vi "Generate_I2C.vi"(8 "Error_In":errorcluster, 10 "Mode":T1, 11 "7Bit_Address_In":refnum<class "7Bit_Address.lvclass">) -> (0 "Error_Out":errorcluster, 3 "7Bit_Address_Out":refnum<class "7Bit_Address.lvclass">)   [LabVIEW 2023, in "7Bit_Address.lvclass"]
uses:
  7Bit_Address.lvclass
  D:/Git/Assignments/SDLC_I2C/SDLC_I2C_LV23V/Class/I2C/I2C.lvclass
  Class/I2C/Controls/Mode.ctl
  Controls/I2C_States.ctl
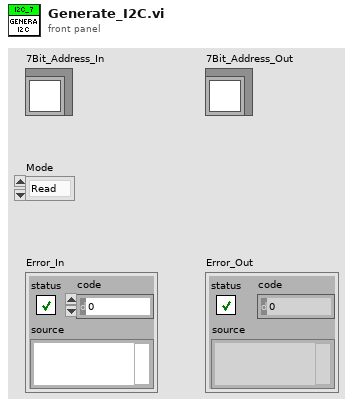
[diagram p1: front panel]
types:
  T1 = typedef "Mode.ctl" = enum16{"Read", "Write"}
  T2 = typedef "I2C_States.ctl" = enum16{"Start", "Byte", "Ack_Nack", "Stop"}
  T3 = typedef "Converted_Data.ctl" = cluster{"Vmin":dbl, "Vmax":dbl, "Input":string, "Off_Set (uS)":dbl, "T_HD_STA (uS)":dbl, "Sample_Per_Us":dbl, "T_HD_DAT (uS)":dbl, "T_SU_DAT (uS)":dbl, "Frequency (kHz)":dbl, "T_SU_STO":dbl, "T_Off (uS)":dbl, "T_On (uS)":dbl, "T_BUF":dbl, "Target_Address":u16, "Register_Address":u8, "Byte_Array":u8[]}
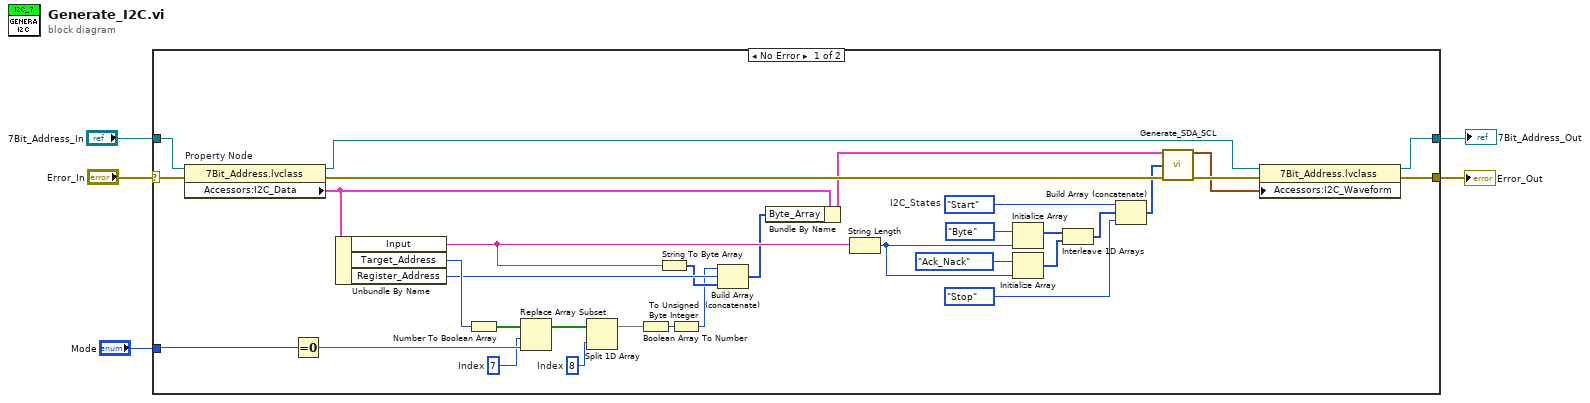
[diagram p0: block diagram]
diagram:
  n1 = case shown="No Error" "Error_In" {
    selector: "Error_In" -> [w37 w40]
    tunnel: [w9 w40] -> w5
    tunnel: [w11 w39] -> w4
    tunnel: "7Bit_Address_In" -> [w26 w39]
    tunnel: "Mode" -> [w22 _]
    frame No Error {
      w6 = 8  # Index
      w19 = 7  # Index
      w35 = I2C_States."Start"  # I2C_States
      n2 = property on="Property Node" class="7Bit_Address.lvclass"(reference=w26, error in=w37) -> (reference out=w25:refnum<class "7Bit_Address.lvclass">, error out=w36:errorcluster, "Accessors:I2C_Data"=w10:T3)
      n3 = Equal To 0?(x=w22) -> (x = 0?=w20:bool)
      n4 = Unbundle By Name(w10) -> ("Input"=w23:string, "Target_Address"=w18:u16, "Register_Address"=w16:u8)
      n5 = Number To Boolean Array(number=w18) -> (Boolean array=w21:bool[])
      n6 = Replace Array Subset(array=w21, new element=w20, index=w19) -> (w8:bool[])
      n7 = Split 1D Array(array=w8, index=w6) -> (first subarray=w7:bool[])  [unwired: 1 out]
      n8 = Boolean Array To Number(Boolean array=w7) -> (number=w17:u32)
      n9 = String To Byte Array(string=w23) -> (unsigned byte array=w15:u8[])
      n10 = To Unsigned Byte Integer(number=w17) -> (unsigned 8bit integer=w14:u8)
      n11 = Build Array (concatenate)(w14, w16, w15) -> (w12:u8[])
      n12 = Bundle By Name(cluster=w10, "Byte_Array"=w12) -> (w13:T3)
      n13 = String Length(string=w23) -> (length=w33:i32)
      n14 = Initialize Array(I2C_States."Byte" ("Enum"), w33) -> (w31:T2[])
      n15 = Initialize Array(I2C_States."Ack_Nack" ("element"), w33) -> (w30:T2[])
      n16 = Interleave 1D Arrays(w31, w30) -> (w29:T2[])
      n17 = Build Array (concatenate)(w35, w29, I2C_States."Stop" ("element")) -> (w27:T2[])
      n18 = call "Generate_SDA_SCL.vi"("Data"=w13, "Data_Sequence"=w27, "Error_In"=w36) -> ("Waveform Graph"=w24:waveform(dbl)[], "Error_Out"=w38:errorcluster)  [unwired: 11 in]
      n19 = property class="7Bit_Address.lvclass"(reference=w25, error in=w38, "Accessors:I2C_Waveform"=w24) -> (reference out=w11:refnum<class "7Bit_Address.lvclass">, error out=w9:errorcluster)
    }
    frame Error {
    }
  }
  "Error_Out" <- w5
  "7Bit_Address_Out" <- w4
